vi "setLevelTriton.vi"(0 "VISA resource name 2":refnum<visa-resource-name>, 1 "Source":T1, 3 "error out 2":errorcluster, 4 "SourceLevel":dbl) -> (5 "VISA resource name":refnum<visa-resource-name>, 6 "String":string, 7 "error out":errorcluster)   [LabVIEW 2021]
uses:
  2450/Source2450.ctl
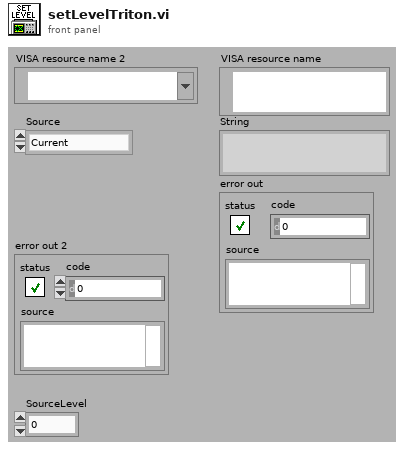
[diagram p1: front panel]
types:
  T1 = typedef "Source2450.ctl" = enum16{"Current", "Voltage"}
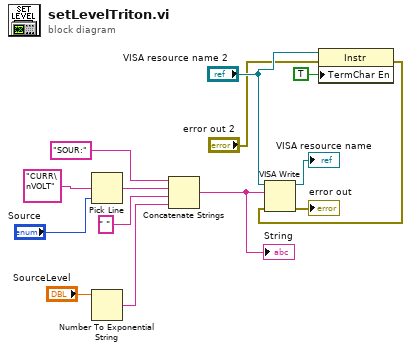
[diagram p0: block diagram]
diagram:
  n1 = Pick Line(multi-line string="CURR\nVOLT", line index="Source") -> (output string=w9:string)  [unwired: 1 in]
  n2 = Number To Exponential String(number="SourceLevel") -> (E-format string=w11:string)  [unwired: 3 in]
  n3 = Concatenate Strings("SOUR:", w9, " " ("string"), w11) -> (w1:string)
  "String" <- w1
  n4 = property class="Instr"(reference="VISA resource name 2", error in="error out 2", "TermChar En"=TRUE ("Message Based Settings:Termination Character Enable")) -> (error out=w2:errorcluster)  [unwired: 1 out]
  n5 = VISA Write(VISA resource name="VISA resource name 2", write buffer=w1, error in (no error)=w2) -> (VISA resource name out=→"VISA resource name":refnum<visa-resource-name>, error out=→"error out":errorcluster)  [unwired: 1 out]
